vi "Read Plot Data.vi"(11 "MCCW ACLR in":refnum<class "MCCW ACLR.lvclass">) -> (2 "Plot Data":cluster{"X-Axis":dbl[], "Y-Axis":dbl[]}[](array[cluster]), 3 "MCCW ACLR out":refnum<class "MCCW ACLR.lvclass">)   [LabVIEW 2020, in "MCCW ACLR.lvclass"]
uses:
  MCCW ACLR.lvclass
  MCCW ACLR.lvclass/MCCW ACLR.ctl
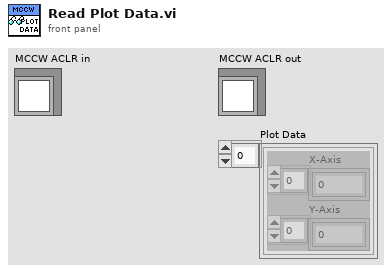
[diagram p1: front panel]
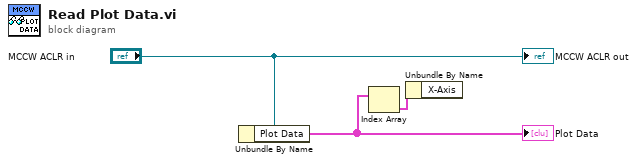
[diagram p0: block diagram]
diagram:
  n1 = Unbundle By Name("MCCW ACLR in") -> ("Plot Data"=w2:cluster{"X-Axis":dbl[], "Y-Axis":dbl[]}[])
  "Plot Data" <- w2
  n2 = Index Array(array=w2) -> (element=w1:cluster{"X-Axis":dbl[], "Y-Axis":dbl[]})  [unwired: 1 in]
  n3 = Unbundle By Name(w1) -> ()  [unwired: 1 out]
  "MCCW ACLR out" <- "MCCW ACLR in"
